vi "Get Frames.vi"(8 "error in (no error)":errorcluster, 10 "Action":T2, 11 "Custom Device reference in":refnum<k24>) -> (0 "error out":errorcluster, 2 "Frame Array":T1[](array[typedef]), 3 "Custom Device reference out":refnum<k24>)   [LabVIEW 2023, in "J1939 System Definition API Support.lvlib"]
uses:
  J1939 System Definition API Support.lvlib
  NationalInstruments.VeriStand.SystemDefinitionAPI
  Types/Remove Frame Action.ctl
  Types/Remove Item - Frame Cluster.ctl
  Addon/Addon Shared/SubVIs/Constants.vi
  <vilib>/NI VeriStand/Custom Device Tools/Custom Device Utility Library/NI VeriStand - Search for All Items by GUID.vi
  <vilib>/NI VeriStand/Custom Device Tools/Custom Device Utility Library/Custom Device Utility Library.lvlib
  Addon/Addon Shared/J1939 Addon Shared.lvlib
  <vilib>/NI VeriStand/Custom Device API/Custom Device API.lvlib
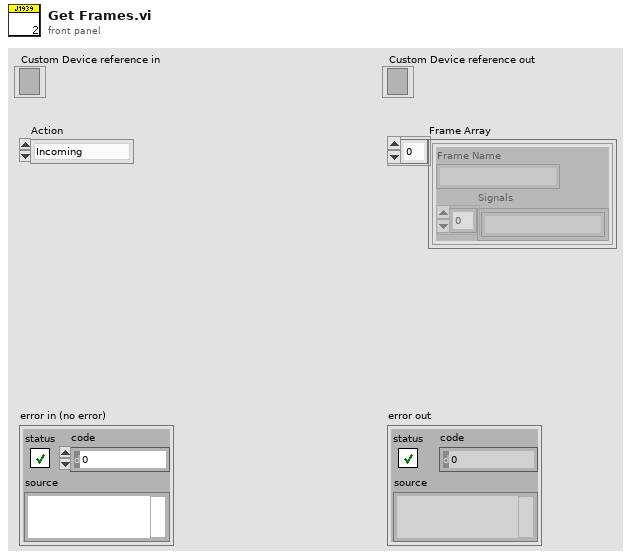
[diagram p1: front panel]
types:
  T1 = typedef "J1939 System Definition API Support.lvlib/Remove Item - Frame Cluster.ctl" = cluster{"Frame Name":string, "Signals":string[]}
  T2 = typedef "J1939 System Definition API Support.lvlib/Remove Frame Action.ctl" = enum16{"Incoming", "Outgoing Event", "Outgoing Cyclic", "Outgoing Cyclic Event"}
  T3 = typedef "Custom Device API.lvlib/Custom Device Item Ref.ctl" = u64
  T4 = typedef "Custom Device API.lvlib/Custom Device Item Info.ctl" = cluster{"Name":string, "Is Channel":bool, "GUID":string, "Is Waveform":bool}
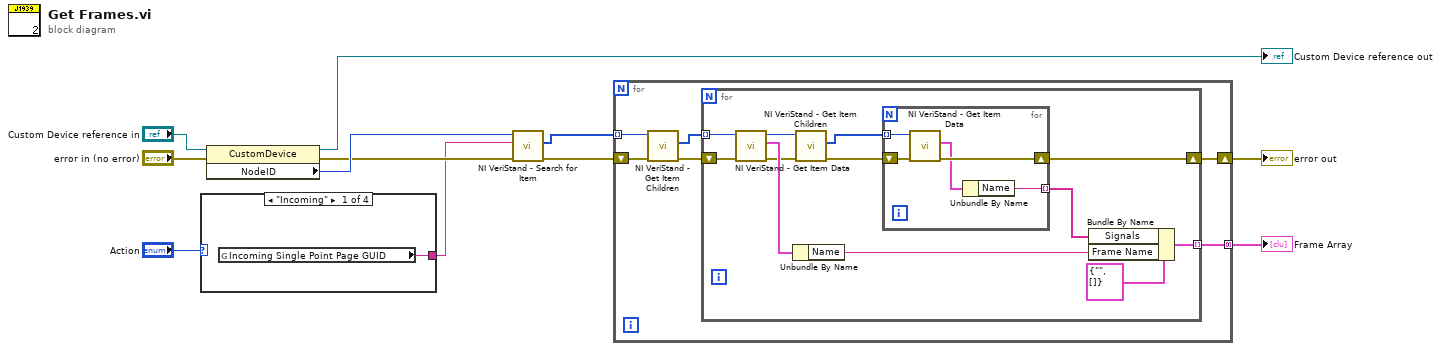
[diagram p0: block diagram]
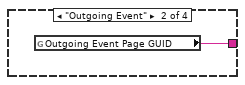
[diagram p2: hidden frame]
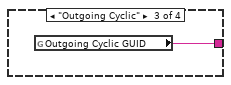
[diagram p3: hidden frame]
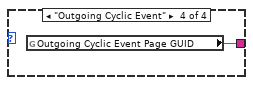
[diagram p4: hidden frame]
diagram:
  n1 = case shown="\"Incoming\"" "Action" {
    tunnel: [w12 w13 w14 w15] -> w1
    frame "Incoming" {
      n2 = global read "Constants.vi" "Incoming Single Point Page GUID"() -> (w12:string)
    }
    frame "Outgoing Event" {
      n3 = global read "Constants.vi" "Outgoing Event Page GUID"() -> (w13:string)
    }
    frame "Outgoing Cyclic" {
      n4 = global read "Constants.vi" "Outgoing Cyclic GUID"() -> (w14:string)
    }
    frame "Outgoing Cyclic Event" {
      n5 = global read "Constants.vi" "Outgoing Cyclic Event Page GUID"() -> (w15:string)
    }
  }
  n6 = property class="CustomDevice"(reference="Custom Device reference in", error in="error in (no error)") -> (reference out=→"Custom Device reference out":refnum<k24>, error out=w10:errorcluster, "NodeID"=w11:u64)
  n7 = call-poly <vilib>:"NI VeriStand - Search for Item.vi"("error in"=w10, "Item GUID"=w1, "Section Ref in"=w11) -> ("error out"=w5:errorcluster, "Item Refs"=w6:T3[])  [unwired: 5 in, 2 out]
  n8 = for {
    tunnel: w6 -> [w21] mode=indexing
    tunnel: [w16] -> w3 mode=concatenating
    shift-right: [w17] -> w4
    shift-left: w5 -> [w20]
    n9 = call <vilib>:"NI VeriStand - Get Item Children.vi"("error in (no error)"=w20, "Item Ref in"=w21) -> ("error out"=w19:errorcluster, "Child Refs"=w18:T3[])  [unwired: 6 in, 2 out]
    n10 = for {
      tunnel: w18 -> [w31] mode=indexing
      shift-right: [w26] -> w17
      shift-left: w19 -> [w33]
      tunnel: [w22] -> w16 mode=indexing
      n11 = call <vilib>:"NI VeriStand - Get Item Data.vi"("error in (no error)"=w33, "Item Ref in"=w31) -> ("error out"=w30:errorcluster, "Item Info"=w32:T4, "Item Ref out"=w29:T3)  [unwired: 6 in, 1 out]
      n12 = Unbundle By Name(w32) -> ("Name"=w24:string)
      n13 = call <vilib>:"NI VeriStand - Get Item Children.vi"("error in (no error)"=w30, "Item Ref in"=w29) -> ("error out"=w27:errorcluster, "Child Refs"=w28:T3[])  [unwired: 6 in, 2 out]
      n14 = for {
        tunnel: w28 -> [w38] mode=indexing
        shift-right: [w36] -> w26
        shift-left: w27 -> [w37]
        tunnel: [w34] -> w23 mode=indexing
        n15 = call <vilib>:"NI VeriStand - Get Item Data.vi"("error in (no error)"=w37, "Item Ref in"=w38) -> ("error out"=w36:errorcluster, "Item Info"=w35:T4)  [unwired: 6 in, 2 out]
        n16 = Unbundle By Name(w35) -> ("Name"=w34:string)
      }
      n17 = Bundle By Name(cluster=T1 {"Frame Name"="", "Signals"=[]} ("Cluster"), "Signals"=w23, "Frame Name"=w24) -> (w22:T1)
    }
  }
  "error out" <- w4
  "Frame Array" <- w3
